vi "RunTimeMenu Wrapper.vi"(8 "error in (no error)":errorcluster, 11 "Node Ptr":u64 format="%.0x") -> (0 "error out":errorcluster)   [LabVIEW 2020, in "AIM ARINC 664 System Explorer.lvlib"]
uses:
  AIM ARINC 664 System Explorer.lvlib
  Includes/afdx_custom_device System Explorer.lvlibp/System Explorer/Implementation/System Explorer Dispatcher/System Explorer Dispatcher.lvclass
  C:/repos/niveristand-aim-afdx-custom-device/Includes/afdx_custom_device System Explorer.lvlibp/System Explorer/Interfaces/System Explorer Dispatcher/System Explorer Dispatcher.lvclass
  Includes/afdx_custom_device System Explorer.lvlibp/System Explorer/Interfaces/System Explorer Dispatcher/System Explorer Dispatcher.lvclass
panel:
  in  "Tag":string
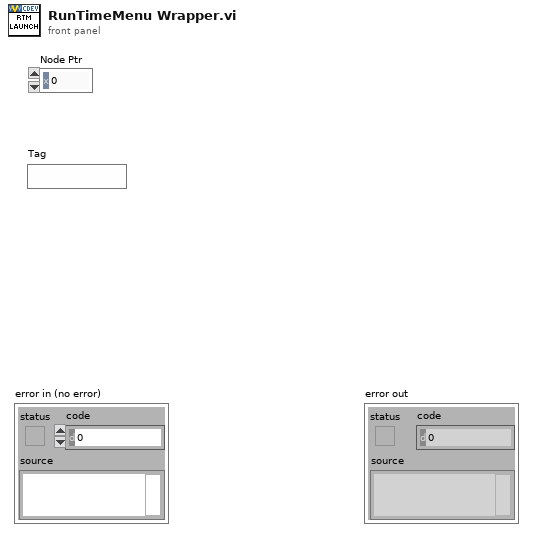
[diagram p1: front panel]
types:
  T1 = typedef "Custom Device API.lvlib/Custom Device Item Ref.ctl" = u64
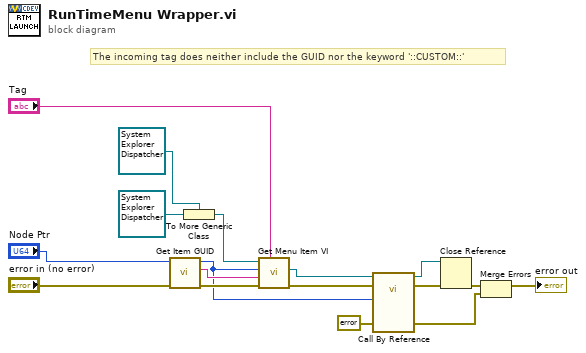
[diagram p0: block diagram]
diagram:
  # "The incoming tag does neither include the GUID nor the keyword '::CUSTOM::'"
  n1 = call "Get Item GUID.vi"("error in (no error)"="error in (no error)", "item in"="Node Ptr") -> ("error out"=w16:errorcluster, "guid"=w15:string, "item out"=w5:T1)  [unwired: 7 in]
  n2 = To More Generic Class(target class=refnum<class "System Explorer Dispatcher.lvclass"> refnum ("afdx_custom_device System Explorer.lvlibp:Interfaces.lvlib:System Explorer Dispatcher.lvclass"), reference=refnum<class "System Explorer Dispatcher.lvclass"> refnum ("afdx_custom_device System Explorer.lvlibp:Implementation.lvlib:System Explorer Dispatcher.lvclass")) -> (generic class reference=w17:refnum<class "System Explorer Dispatcher.lvclass">)
  n3 = call-dynamic "Get Menu Item VI.vi"("Menu Item"="Tag", "error in (no error)"=w16, "GUID"=w15, "Item Ref"=w5, "System Explorer Dispatcher in"=w17) -> ("error out"=w13:errorcluster, "menu item reference"=w14:refnum<vi>)  [unwired: 4 in, 1 out]
  n4 = call-by-ref "?"(reference=w14, error in=w13, 8:"error in (no error)"=errorcluster {"status"=FALSE, "code"=0, "source"=""} ("error in"), "Node Ptr"=w5) -> (reference out=w9:refnum<vi>, error out=w10:errorcluster, 0:"error out"=w3:errorcluster)  [unwired: 9 in]
  n5 = Close Reference(reference=w9, error in (no error)=w10) -> (error out=w8:errorcluster)
  n6 = Merge Errors(w8, w3) -> (→"error out":errorcluster)
